vi "Sweep BL Fine.vi"(8 "error in (no error)":errorcluster, 9 "Sweep outfile":path, 10 "addr":i32, 11 "instrument handle":refnum<k15>) -> (0 "error out":errorcluster, 1 "final current (A)":dbl, 2 "final resistance (ohm)":dbl, 3 "instrument handle out":refnum<k15>)   [LabVIEW 2018]
uses:
  <vilib>/Utility/file.llb/Write Delimited Spreadsheet (DBL).vi
panel:
  out "i":i32
  out "PW":i32
  out "BL voltage (V)":dbl
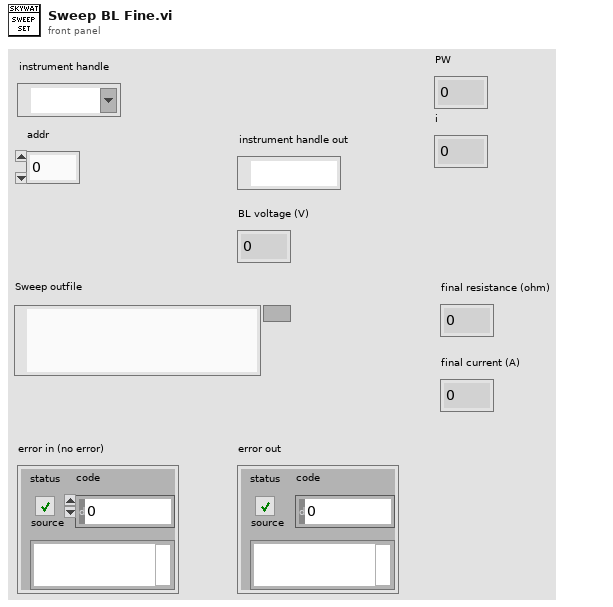
[diagram p1: front panel]
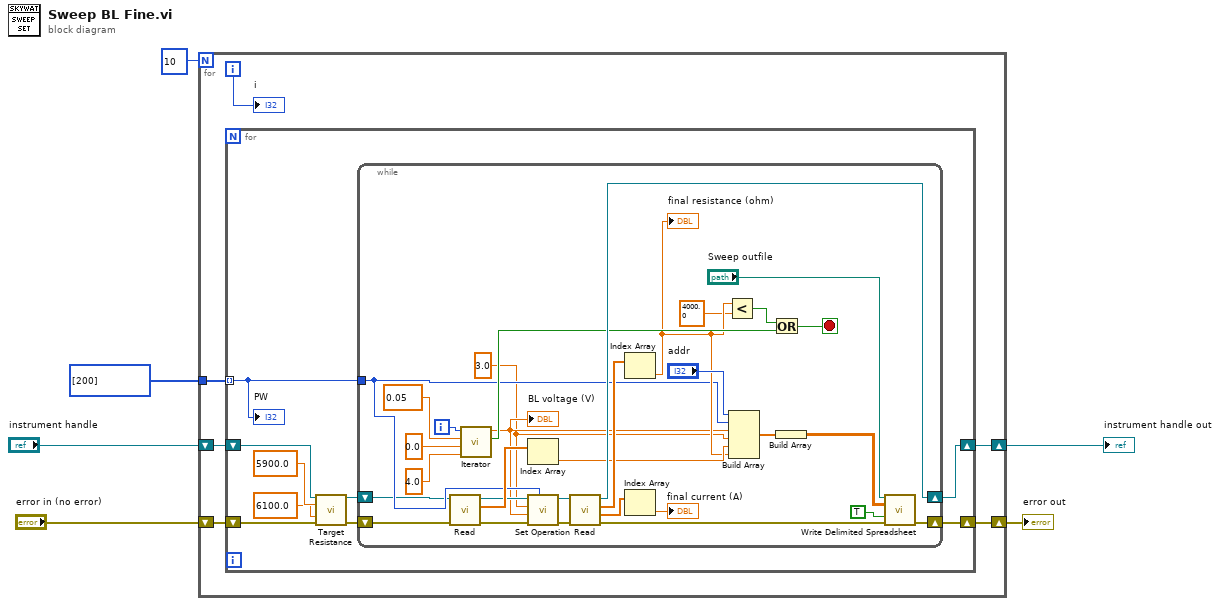
[diagram p0: block diagram]
diagram:
  n1 = for {
    N: 10 -> [_]
    tunnel: i32[] [200] -> [w8]
    shift-right: [w12] -> w6
    shift-left: "instrument handle" -> [w11]
    shift-right: [w9] -> w3
    shift-left: "error in (no error)" -> [w10]
    i -> [w7]
    n2 = for {
      shift-right: [w21] -> w12
      shift-left: w11 -> [w18]
      shift-right: [w20] -> w9
      shift-left: w10 -> [w15]
      tunnel: w8 -> [w19] mode=indexing
      n3 = call "Target Resistance.vi"("instrument handle"=w18, "Lower resistance (ohm)"=5900.0, "Upper resistance (ohm)"=6100.0, "error in (no error)"=w15) -> ("instrument handle out"=w17:refnum<k15>, "error out"=w16:errorcluster)  [unwired: 4 in, 6 out]
      n4 = while {
        shift-right: [w44] -> w21
        shift-left: w17 -> [w27]
        shift-right: [w47] -> w20
        shift-left: w16 -> [w26]
        tunnel: w19 -> [w29]
        i -> [w23]
        stop <- w38 stop-if-true
        w22 = 3.0 ("Numeric Control")
        n5 = call "Read.vi"("error in (no error)"=w26, "instrument handle"=w27) -> ("error out"=w32:errorcluster, "resistances (ohm)"=w40:dbl[], "instrument handle out"=w33:refnum<k15>)  [unwired: 6 in, 1 out]
        n6 = call "Iterator.vi"("Final Value"=4.0 ("y"), "Initial Value"=0.0 ("y"), "Step"=0.05 ("x"), "i"=w23) -> ("End Loop"=w37:bool, "Current Value"=w25:dbl)  [unwired: 6 in]
        "BL voltage (V)" <- w25
        n7 = Index Array(array=w40) -> (element=w39:dbl)  [unwired: 1 in]
        n8 = call "Set Operation.vi"("PW"=w29, "error in (no error)"=w32, "BLV"=w25, "WLV"=w22, "instrument handle"=w33) -> ("error out"=w31:errorcluster, "instrument handle out"=w30:refnum<k15>)  [unwired: 5 in]
        n9 = call "Read.vi"("error in (no error)"=w31, "instrument handle"=w30) -> ("error out"=w45:errorcluster, "currents (A)"=w42:dbl[], "resistances (ohm)"=w43:dbl[], "instrument handle out"=w44:refnum<k15>)  [unwired: 6 in]
        n10 = Index Array(array=w43) -> (element=w36:dbl)  [unwired: 1 in]
        "final resistance (ohm)" <- w36
        n11 = Index Array(array=w42) -> (element=→"final current (A)":dbl)  [unwired: 1 in]
        n12 = Less?(x=w36, y=4000.0 ("x")) -> (x < y?=w34:bool)
        n13 = Build Array("addr", w29, w25, w22, w39, w36) -> (w49:dbl[])
        n14 = Or(x=w34, y=w37) -> (x .or. y?=w38:bool)
        n15 = Build Array(w49) -> (w50:dbl[][])
        n16 = call-poly <vilib>:"Write Delimited Spreadsheet.vi"("file path (dialog if empty)"="Sweep outfile", "2D data"=w50, "append to file? (new file:F)"=TRUE, "error in (no error)"=w45) -> ("error out"=w47:errorcluster)  [unwired: 10 in, 1 out]
      }
      "PW" <- w19
    }
    "i" <- w7
  }
  "error out" <- w3
  "instrument handle out" <- w6
